vi "Write AFG Resource.vi"(8 "error in (no error)":errorcluster, 9 "Simulated AFG":bool, 10 "AFG resource name":refnum<visa-resource-name>, 11 "Unit_Test_AFG in":refnum<class "Unit_Test_AFG.lvclass">) -> (0 "error out":errorcluster, 3 "Unit_Test_AFG out":refnum<class "Unit_Test_AFG.lvclass">)   [LabVIEW 2020, in "Unit_Test_AFG.lvlib" / "Unit_Test_AFG.lvclass"]
uses:
  Unit_Test_AFG.lvclass
  Unit_Test_AFG.lvclass/Unit_Test_AFG.ctl
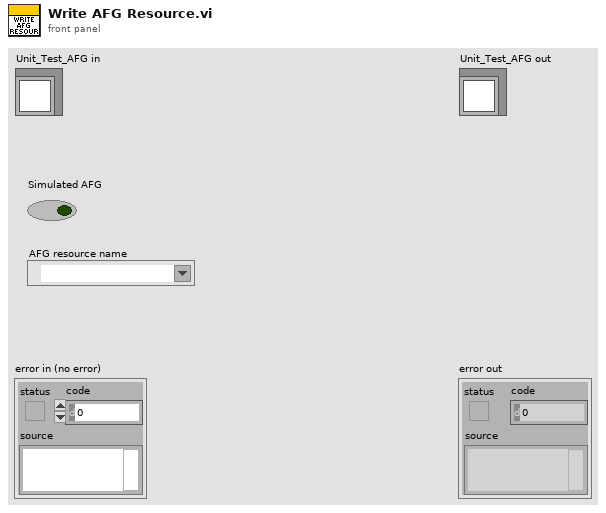
[diagram p1: front panel]
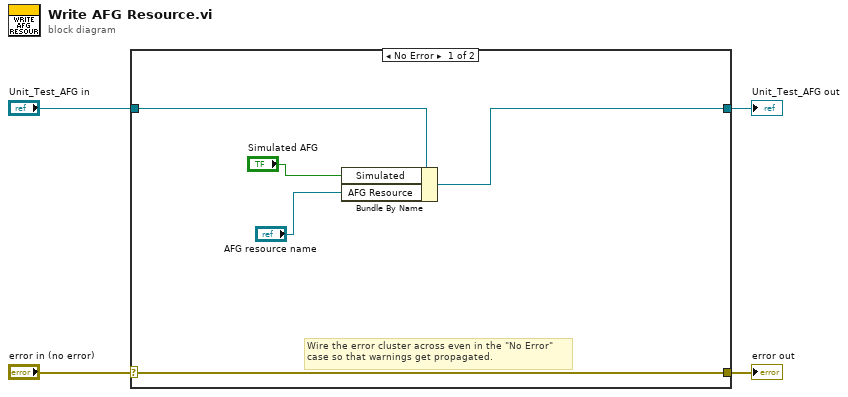
[diagram p0: block diagram]
diagram:
  n1 = case shown="No Error" "error in (no error)" {
    selector: "error in (no error)" -> [w9 w11]
    tunnel: [w9 w11] -> w3
    tunnel: [w5 w10] -> w1
    tunnel: "Unit_Test_AFG in" -> [w8 w10]
    frame No Error {
      # "Wire the error cluster across even in the \"No Error\"\ncase so that warnings get propagated."
      n2 = Bundle By Name(cluster=w8, "Simulated"="Simulated AFG", "AFG Resource"="AFG resource name") -> (w5:refnum<class "Unit_Test_AFG.lvclass">)
    }
    frame Error {
    }
  }
  "error out" <- w3
  "Unit_Test_AFG out" <- w1
